vi "ListSEQFile.vi"(11 "Path":string) -> (3 "SEQ Path":string[](array[string]))   [LabVIEW 2020]
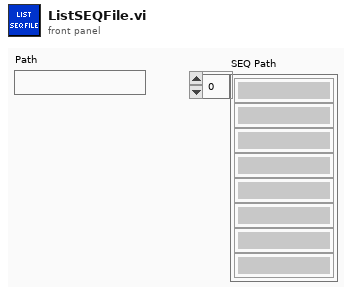
[diagram p1: front panel]
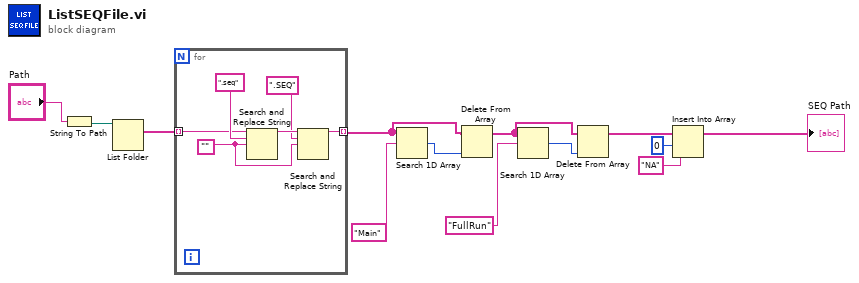
[diagram p0: block diagram]
diagram:
  n1 = String To Path(string="Path") -> (path=w13:path)
  n2 = List Folder(path=w13) -> (filenames=w12:string[])  [unwired: 3 in, 3 out]
  n3 = for {
    tunnel: w12 -> [w18] mode=indexing
    tunnel: [w16] -> w9 mode=indexing
    w15 = ""
    n4 = Search and Replace String(input string=w18, search string=".seq", replace string=w15) -> (result string=w17:string)  [unwired: 5 in, 3 out]
    n5 = Search and Replace String(input string=w17, search string=".SEQ", replace string=w15) -> (result string=w16:string)  [unwired: 5 in, 3 out]
  }
  n6 = Search 1D Array(1D array=w9, element="Main") -> (index of element=w8:i32)  [unwired: 1 in]
  n7 = Delete From Array(array=w9, index=w8) -> (array with subset deleted=w5:string[])  [unwired: 1 in, 1 out]
  n8 = Search 1D Array(1D array=w5, element="FullRun") -> (index of element=w6:i32)  [unwired: 1 in]
  n9 = Delete From Array(array=w5, index=w6) -> (array with subset deleted=w4:string[])  [unwired: 1 in, 1 out]
  n10 = Insert Into Array(array=w4, index=0, new element="NA" ("new element/subarray")) -> (→"SEQ Path":string[])
